vi "Callback_Get Control.vi"(4 "context in":variant, 5 "objref":refnum<vi>) -> (1 "context out":variant, 2 "traverse flags":i32)   [LabVIEW 2018, in "NISAST VI Scripting.lvlib" / "VI.lvlib" / "Front Panel.lvlib"]
uses:
  Front Panel.lvlib
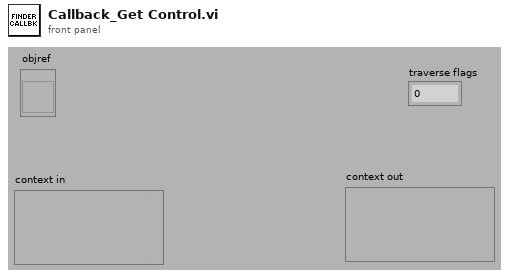
[diagram p1: front panel]
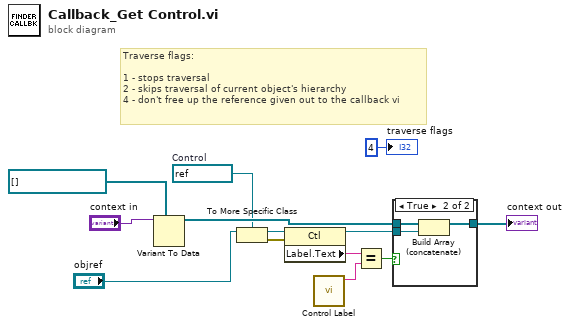
[diagram p0: block diagram]
diagram:
  w7 = refnum<vi> refnum  # Control
  # "Traverse flags:\n\n1\t- stops traversal \n2\t- skips traversal of current object's hierarchy\n4 - don't free up the reference given out to the callback vi"
  n1 = Variant To Data(type=refnum<vi>[] [], Variant="context in") -> (data=w11:refnum<vi>[])  [unwired: 1 in, 1 out]
  n2 = To More Specific Class(target class=w7, reference="objref") -> (specific class reference=w6:refnum<vi>, error out=w4:errorcluster)  [unwired: 1 in]
  n3 = property class="Ctl"(reference=w6, error in=w4) -> (reference out=w5:refnum<vi>, "Label.Text"=w3:string)  [unwired: 1 out]
  n4 = call "Control Label.vi"() -> ("label out"=w2:string)  [unwired: 3 in, 8 out]
  n5 = Equal?(x=w3, y=w2) -> (x = y?=w1:bool)
  n6 = case shown="True" w1 {
    tunnel: w11 -> [w14 w17]
    tunnel: [w14 w16] -> w10
    tunnel: w5 -> [_ w15]
    frame False {
    }
    frame True {
      n7 = Build Array (concatenate)(w17, w15) -> (w16:refnum<vi>[])
    }
  }
  "context out" <- w10
  "traverse flags" <- 4 ("Traverse Flags")
